vi "GetType.vi"(8 "error in (no error)":errorcluster, 11 "Log Data Msg":refnum<class "Log Data Msg.lvclass">) -> (0 "error out":errorcluster, 2 "Data Sample":variant, 3 "Log Data Msg":refnum<class "Log Data Msg.lvclass">)   [LabVIEW 2016, in "LS218.lvlib" / "Log Data Msg.lvclass"]
uses:
  Log Data Msg.lvclass
  Log Data Msg.lvclass/Log Data Msg.ctl
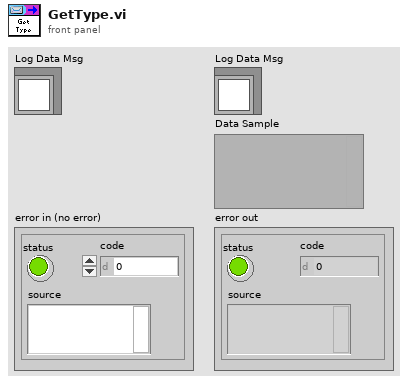
[diagram p1: front panel]
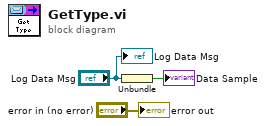
[diagram p0: block diagram]
diagram:
  n1 = Unbundle("Log Data Msg") -> (→"Data Sample":bool)
  "error out" <- "error in (no error)"
  "Log Data Msg" <- "Log Data Msg"
